vi "ziPollDataExDemodTime.vi"(8 "error in":errorcluster, 9 "recording time (1) [s]":dbl=1.0, 10 "SubscribepathArray":string[](array[string])=["demods/0/sample"], 11 "Handle In":T2 {"Handle" format="0x%08x"; "Conn" format="0x%08x"}) -> (0 "error out":errorcluster, 2 "Demod Sample Out":T1[](array[typedef]) {"Aux In 1 (V)" format="%#_5p"; "Aux In 0 (V)" format="%#_5p"; "X (Vrms)" format="%#_5p"; "Y (Vrms)" format="%#_5p"; "Osc Phase (rad)" format="%#.3g"}, 3 "Handle Out":T2 {"Handle" format="0x%08x"; "Conn" format="0x%08x"})   [LabVIEW 2018, in "Zurich Instruments LabOne.lvlib"]
doc: "This vi polls <b>Demod data</b> from a previously subscriped demod path for a given <b>recording time</b>."
uses:
  Zurich Instruments LabOne.lvlib
  ziTypeDemodSampleEx.ctl
  ziGetEventDemodSample.vi
  Utility/ziTicksToS_vector.vi
  ziTypeHandle.ctl
panel:
  out "?":i32
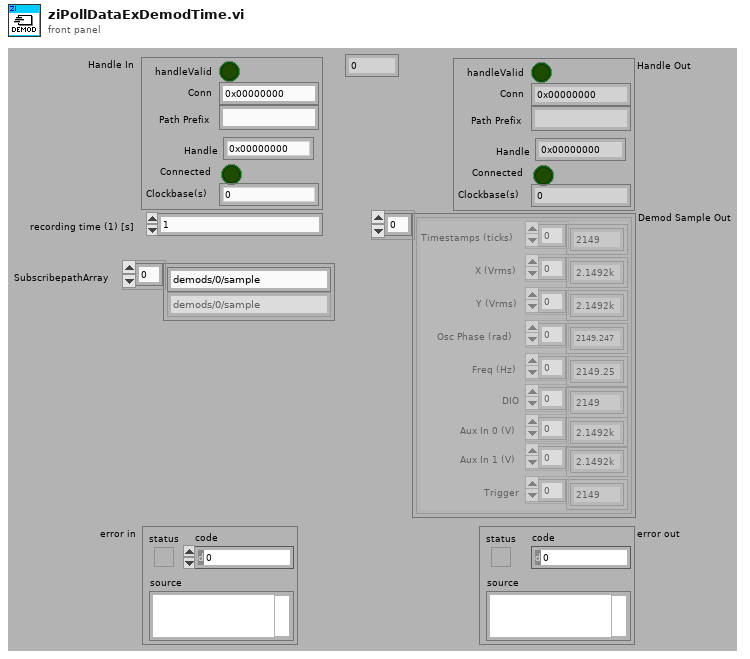
[diagram p1: front panel]
types:
  T1 = typedef "Zurich Instruments LabOne.lvlib/ziTypeDemodSampleEx.ctl" = cluster{"Timestamps (ticks)":u64[], "X (Vrms)":dbl[], "Y (Vrms)":dbl[], "Osc Phase (rad)":dbl[], "Freq (Hz)":dbl[], "DIO":u32[], "Aux In 0 (V)":dbl[], "Aux In 1 (V)":dbl[], "Trigger":u32[]}
  T2 = typedef "Zurich Instruments LabOne.lvlib/ziTypeHandle.ctl" = cluster{"handleValid":bool, "Conn":u64, "Path Prefix":string, "Handle":u64, "Connected":bool, "Clockbase(s)":dbl}
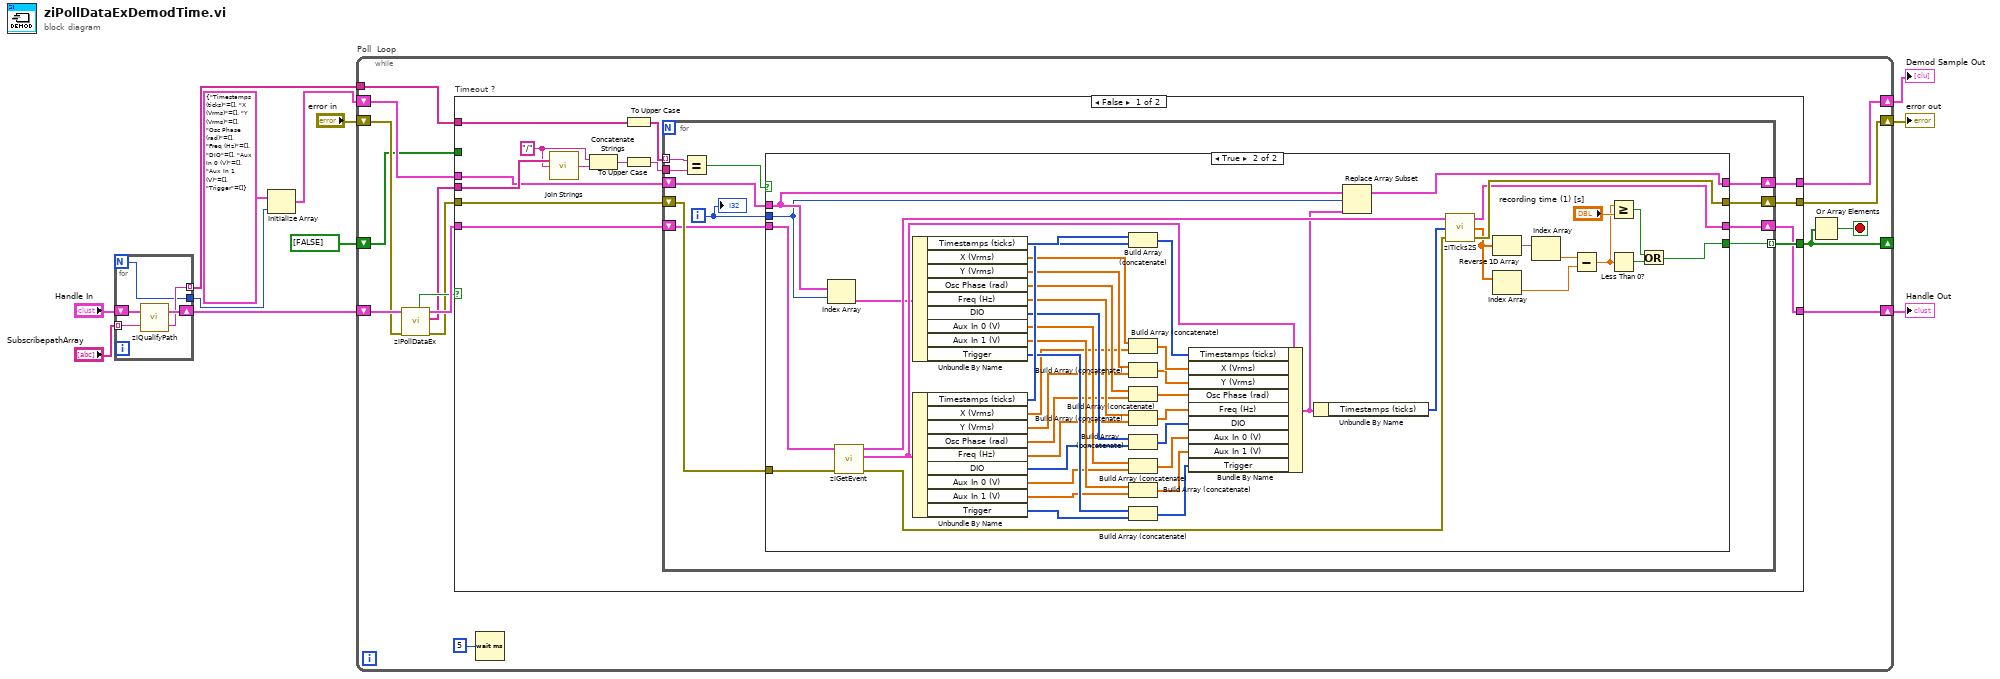
[diagram p0: block diagram]
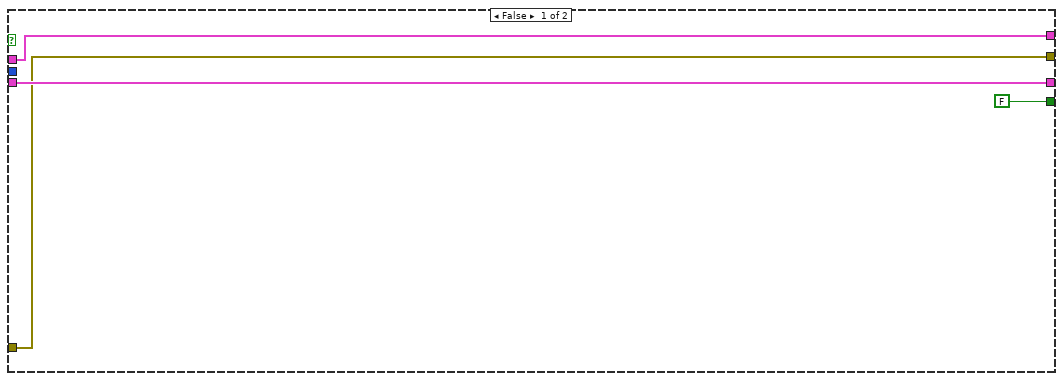
[diagram p2: hidden frame]
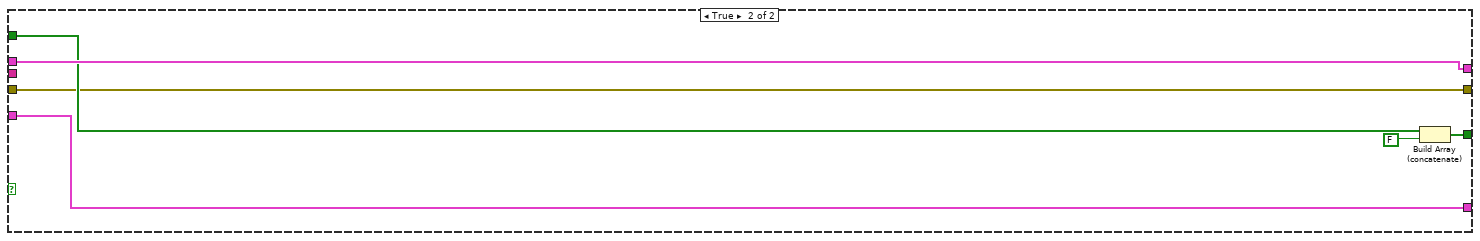
[diagram p3: hidden frame]
diagram:
  n1 = for {
    N -> [w13]
    tunnel: "SubscribepathArray" -> [w15] mode=indexing
    tunnel: [w14] -> w6 mode=indexing
    shift-right: [w16] -> w8
    shift-left: "Handle In" -> [w17]
    tunnel: [w13] -> w3
    n2 = call "ziQualifyPath.vi"("Path In"=w15, "Handle In"=w17) -> ("Path Out"=w14:string, "Handle Out"=w16:T2)
  }
  n3 = Initialize Array(T1 {"Timestamps (ticks)"=[], "X (Vrms)"=[], "Y (Vrms)"=[], "Osc Phase (rad)"=[], "Freq (Hz)"=[], "DIO"=[], "Aux In 0 (V)"=[], "Aux In 1 (V)"=[], "Trigger"=[]} ("Demod Sample Out"), w3) -> (w2:T1[])
  n4 = while "Poll  Loop" {
    shift-right: [w21] -> w12
    shift-left: w8 -> [w26]
    shift-right: [w29] -> w11
    shift-left: "error in" -> [w25]
    tunnel: w6 -> [w24]
    shift-right: [w23] -> w5
    shift-left: w2 -> [w22]
    shift-right: [w19] -> _
    shift-left: bool[] [FALSE] -> [w20]
    stop <- w18 stop-if-true
    n5 = call "ziPollDataEx.vi"("error in"=w25, "Handle In"=w26) -> ("error out"=w30:errorcluster, "PathArray"=w28:string[], "Handle Out"=w32:T2, "Timed Out"=w31:bool)  [unwired: 2 in, 4 out]
    n6 = case "Timeout ?" shown="False" w31 {
      tunnel: w32 -> [w35 w115]
      tunnel: w30 -> [w46 w111]
      tunnel: [w45 w111] -> w29
      tunnel: w28 -> [w43 _]
      tunnel: w24 -> [w39 _]
      tunnel: [w37 w113] -> w19
      tunnel: [w33 w116] -> w23
      tunnel: w22 -> [w36 w116]
      tunnel: [w34 w115] -> w21
      tunnel: w20 -> [_ w114]
      frame False {
        w42 = "/" ("Separator (,)")
        n7 = call <vilib>:"Join Strings.vi"("Separator (,)"=w42, "Strings In"=w43) -> ("String"=w44:string)  [unwired: 1 in]
        n8 = Concatenate Strings(w42, w44) -> (w38:string)
        n9 = To Upper Case(1:w39) -> (0:w40:string[])
        n10 = To Upper Case(1:w38) -> (0:w41:string)
        n11 = for {
          tunnel: w41 -> [w54]
          tunnel: w40 -> [w53] mode=indexing
          tunnel: [w52] -> w37 mode=indexing
          shift-right: [w55] -> w45
          shift-left: w46 -> [w56]
          shift-right: [w57] -> w34
          shift-left: w35 -> [w50]
          shift-right: [w49] -> w33
          shift-left: w36 -> [w48]
          i -> [w47]
          n12 = Equal?(x=w53, y=w54) -> (x = y?=w51:bool)
          n13 = case shown="True" w51 {
            tunnel: w50 -> [w61 w110]
            tunnel: [w61 w77] -> w57
            tunnel: w56 -> [w60 w109]
            tunnel: [w60 w78] -> w55
            tunnel: [FALSE w68] -> w52
            tunnel: [w58 w66] -> w49
            tunnel: w48 -> [w58 w63]
            tunnel: w47 -> [_ w62]
            frame False {
            }
            frame True {
              n14 = Index Array(array=w63, index=w62) -> (element=w64:T1)
              n15 = call-poly "ziGetEvent.vi"("Error In"=w109, "Handle In"=w110) -> ("Error Out"=w80:errorcluster, "Demod Sample Out"=w67:T1, "Handle Out"=w81:T2)  [unwired: 7 in]
              n16 = Unbundle By Name(w64) -> ("Timestamps (ticks)"=w108:u64[], "X (Vrms)"=w105:dbl[], "Y (Vrms)"=w104:dbl[], "Osc Phase (rad)"=w103:dbl[], "Freq (Hz)"=w102:dbl[], "DIO"=w97:u32[], "Aux In 0 (V)"=w96:dbl[], "Aux In 1 (V)"=w95:dbl[], "Trigger"=w94:u32[])
              n17 = Unbundle By Name(w67) -> ("Timestamps (ticks)"=w107:u64[], "X (Vrms)"=w89:dbl[], "Y (Vrms)"=w88:dbl[], "Osc Phase (rad)"=w87:dbl[], "Freq (Hz)"=w86:dbl[], "DIO"=w85:u32[], "Aux In 0 (V)"=w84:dbl[], "Aux In 1 (V)"=w83:dbl[], "Trigger"=w82:u32[])
              n18 = Build Array (concatenate)(w108, w107) -> (w106:u64[])
              n19 = Build Array (concatenate)(w105, w89) -> (w101:dbl[])
              n20 = Build Array (concatenate)(w104, w88) -> (w100:dbl[])
              n21 = Build Array (concatenate)(w103, w87) -> (w99:dbl[])
              n22 = Build Array (concatenate)(w102, w86) -> (w98:dbl[])
              n23 = Build Array (concatenate)(w97, w85) -> (w93:u32[])
              n24 = Build Array (concatenate)(w96, w84) -> (w92:dbl[])
              n25 = Build Array (concatenate)(w95, w83) -> (w91:dbl[])
              n26 = Build Array (concatenate)(w94, w82) -> (w90:u32[])
              n27 = Bundle By Name(cluster=w67, "Timestamps (ticks)"=w106, "X (Vrms)"=w101, "Y (Vrms)"=w100, "Osc Phase (rad)"=w99, "Freq (Hz)"=w98, "DIO"=w93, "Aux In 0 (V)"=w92, "Aux In 1 (V)"=w91, "Trigger"=w90) -> (w65:T1)
              n28 = Unbundle By Name(w65) -> ("Timestamps (ticks)"=w79:u64[])
              n29 = Replace Array Subset(array=w63, new element=w65, index=w62) -> (w66:T1[])
              n30 = call-poly "ziTicks2S.vi"("Error In"=w80, "Timestamp (ticks)"=w79, "Handle In"=w81) -> ("Error Out"=w78:errorcluster, "Timestamp(s)"=w75:dbl[], "Handle Out"=w77:T2)
              n31 = Reverse 1D Array(array=w75) -> (reversed array=w76:dbl[])
              n32 = Index Array(array=w75) -> (element=w73:dbl)  [unwired: 1 in]
              n33 = Index Array(array=w76) -> (element=w74:dbl)  [unwired: 1 in]
              n34 = Subtract(x=w74, y=w73) -> (x-y=w70:dbl)
              n35 = Greater Or Equal?(x=w70, y="recording time (1) [s]") -> (x >= y?=w69:bool)
              n36 = Less Than 0?(x=w70) -> (x < 0?=w71:bool)
              n37 = Or(x=w69, y=w71) -> (x .or. y?=w68:bool)
            }
          }
          "?" <- w47
        }
      }
      frame True {
        n38 = Build Array (concatenate)(w114, FALSE) -> (w113:bool[])
      }
    }
    n39 = Wait (ms)(milliseconds to wait=u32 5) -> ()  [unwired: 1 out]
    n40 = Or Array Elements(Boolean array=w19) -> (logical OR=w18:bool)
  }
  "Handle Out" <- w12
  "error out" <- w11
  "Demod Sample Out" <- w5
